vi "Test Restore Point.vi"() -> ()   [LabVIEW 2020, in "Test Executive.lvlib"]
uses:
  <vilib>/gpm_packages/@cs/test-executive/Source/Test Executive/Test Executive.lvlib
  <vilib>/gpm_packages/@cs/test-executive/Source/Test Executive/TestExecutive/Test Executive.lvclass
  C:/Program Files/National Instruments/LabVIEW 2020/vi.lib/gpm_packages/@cs/test-executive/Source/Test Executive/ITestExecutive/ITest Executive.lvclass
  <vilib>/gpm_packages/@cs/test-executive/Source/Test Executive/Executioner/Executioner.lvclass
  866dfd19-2fef-4b99-8a4a-1d31d88e504e.vi
  55b154ae-6d03-47ed-abc2-d28db7feda01.vi
  8564ab31-dd3a-4968-8861-3b4339f4920d.vi
  9b79477b-4d99-41b4-a2fb-9df7ea8afb31.vi
  95889fa5-b0fb-411b-bc35-b648c597537f.vi
  6decda23-fb0c-4e77-ad71-e1f71655b843.vi
  71592cda-0d0e-4ea7-b138-086424aed341.vi
  0583369c-d912-4d49-be3f-0b23069dcf00.vi
  bffa5b7c-ecbc-40cd-a0d5-f9da2a76cf50.vi
  <vilib>/Utility/error.llb/Error Cluster From Error Code.vi
  <vilib>/gpm_packages/@cs/test-executive/Source/Test Executive/ITestExecutive/ITest Executive.lvclass
  <vilib>/gpm_packages/@cs/test-executive/Source/Test Executive/TestExecutive Ref/TestExecutive Ref.lvclass
  c9edba23-499d-4d6b-bf99-6c37c6a75b36.vi
  b25967a6-4fd7-4e76-b6fa-60230ccf68d8.vi
panel:
  out "After Restore Run":string[](array[string])
  in  "Stop final run":bool
  out "Final Run classes":string
  out "Restore Traverse":string[](array[string])
  out "Restore Traverse Classes":string
  in  "stop restore":bool
  out "First Run Array":string[](array[string])
  out "Class":string
  out "Tag":i32
  out "Name":string
  out "Attribute 2":i32
  out "class name":string
  in  "stop":bool
  out "error out":errorcluster
  in  "Test Exec":string(tree)
  out "Pointer?":bool
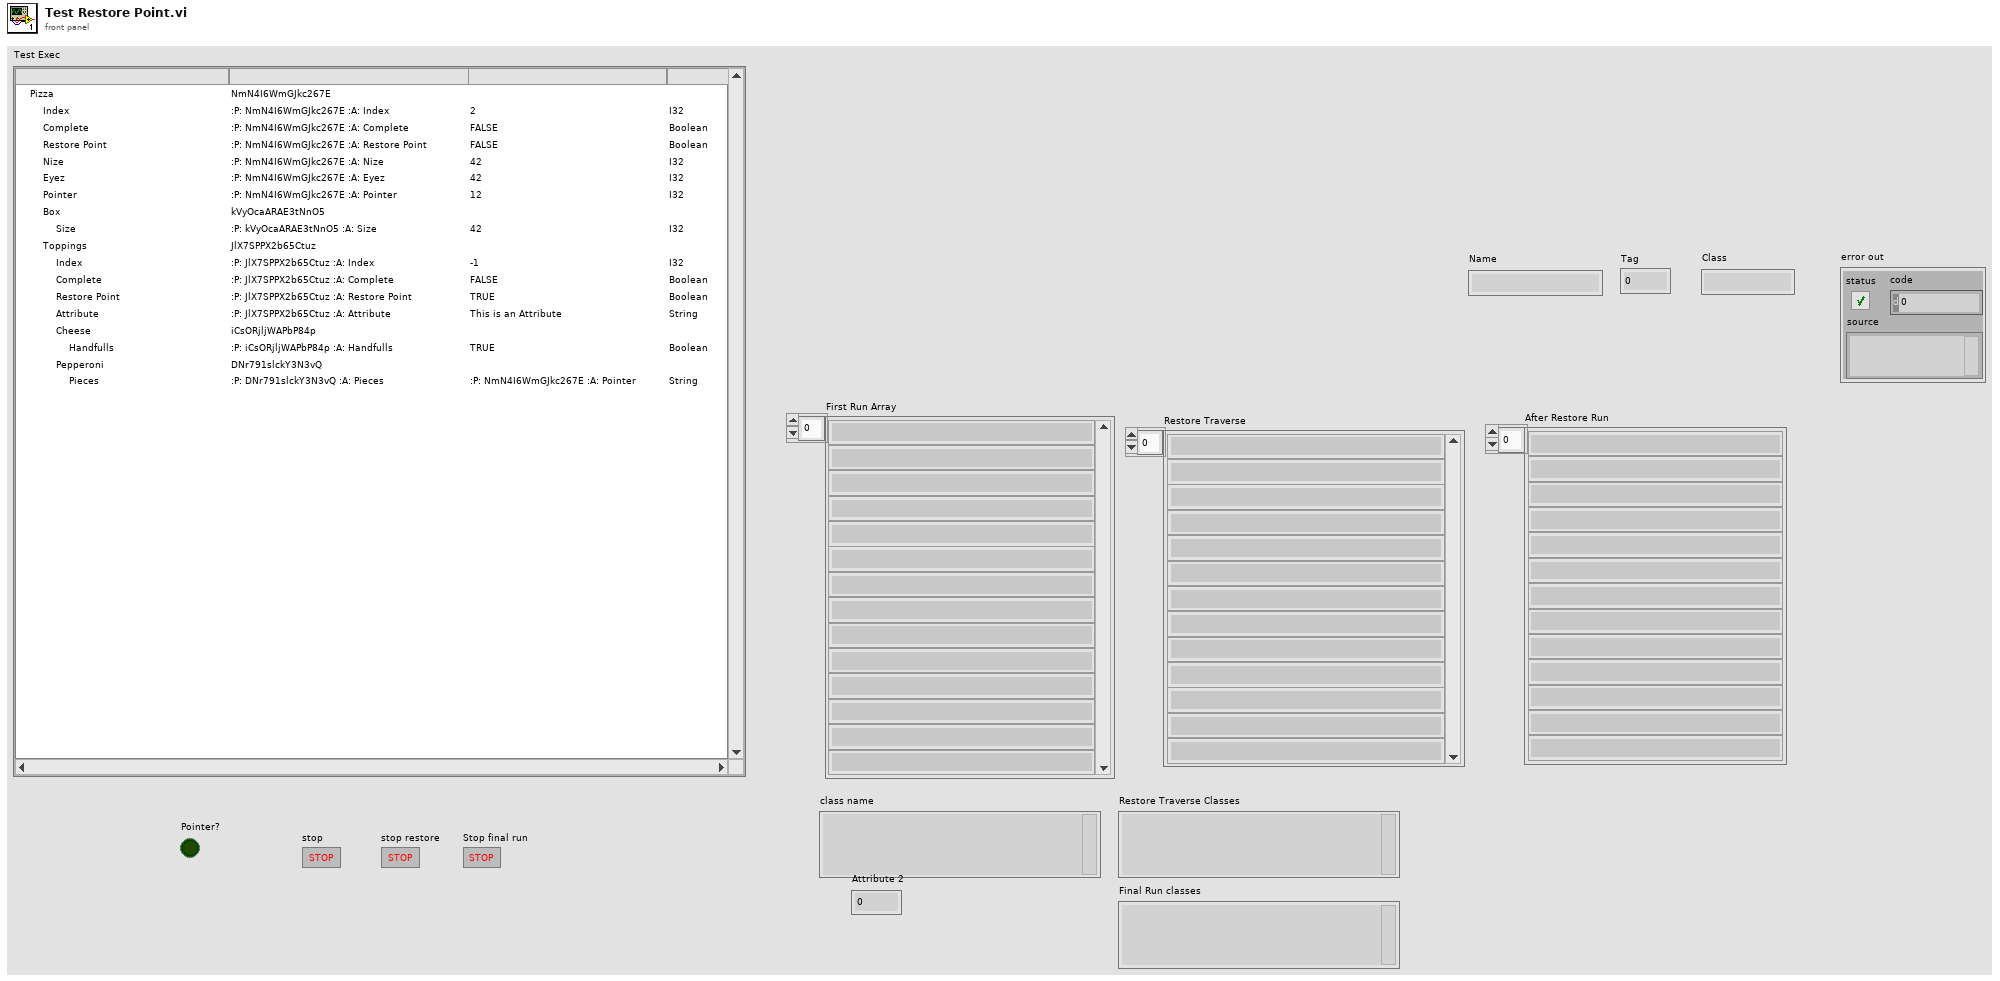
[diagram p1: front panel]
types:
  T1 = cluster{"Left Cell String":string, "Child Text":string[], "Child Tag":string, "Item Indent":i32, "Child Only?":bool, "Glyph Index":i32}[]
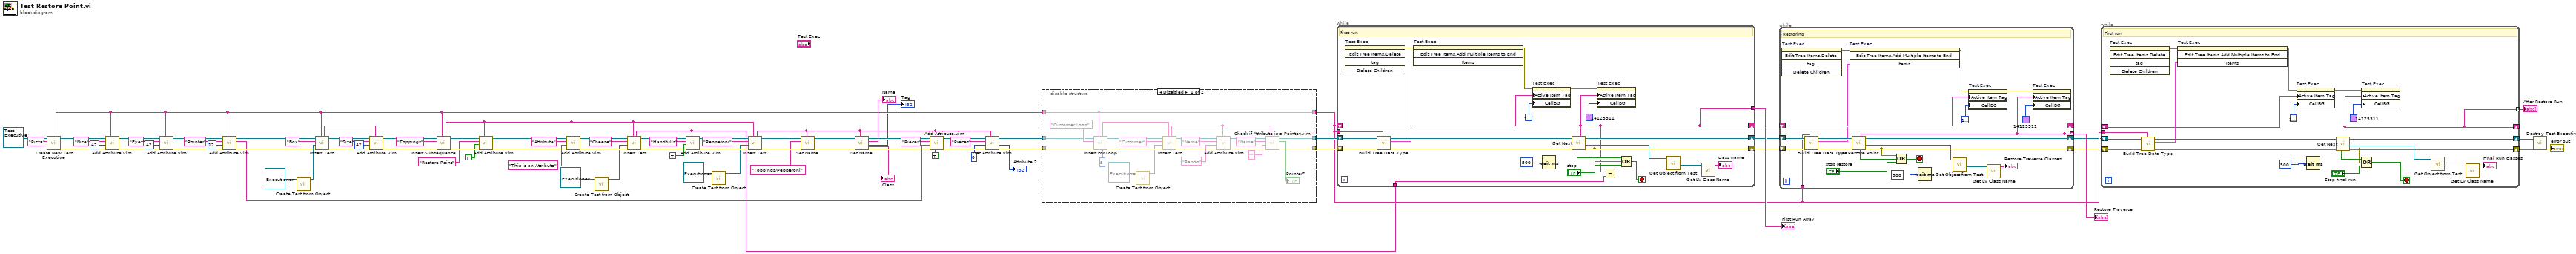
[diagram p0: block diagram]
diagram:
  n1 = call <vilib>:"Create New Test Executive.vi"("Name"="Pizza", "Test Executive"=refnum<class "Test Executive.lvclass"> refnum ("Test Executive.lvlib:Test Executive.lvclass")) -> ("error out"=w56:errorcluster, "Test Executive Ref"=w57:refnum<data-value>, "Test Executive ID out"=w43:string)  [unwired: 7 in]
  n2 = call "Add Attribute.vim"("ID"=w43, "error in (no error)"=w56, "Attribute"=42, "Attribute Name"="Nize", "Test Executive Ref"=w57) -> ("error out"=w52:errorcluster, "Test Executive Ref out"=w53:refnum<data-value>)  [unwired: 3 in, 2 out]
  n3 = call "Add Attribute.vim"("ID"=w43, "error in (no error)"=w52, "Attribute"=42, "Attribute Name"="Eyez", "Test Executive Ref"=w53) -> ("error out"=w47:errorcluster, "Test Executive Ref out"=w45:refnum<data-value>)  [unwired: 3 in, 2 out]
  n4 = call "Add Attribute.vim"("ID"=w43, "error in (no error)"=w47, "Attribute"=12, "Attribute Name"="Pointer", "Test Executive Ref"=w45) -> ("error out"=w46:errorcluster, "Attribute ID out"=w42:string, "Test Executive Ref out"=w44:refnum<data-value>)  [unwired: 3 in, 1 out]
  n5 = call <vilib>:"Create Test from Object.vi"("Test"=refnum<class "Executioner.lvclass"> refnum ("Test Executive.lvlib:Executioner.lvclass")) -> ("Test"=w62:refnum<class "Executioner.lvclass">)  [unwired: 10 in]
  n6 = call <vilib>:"Insert Test.vi"("Parent ID"=w43, "error in (no error)"=w46, "Test"=w62, "Name"="Box", "Test Executive Ref"=w44) -> ("error out"=w70:errorcluster, "Test Executive Ref out"=w85:refnum<data-value>, "Unique ID out"=w84:string)  [unwired: 3 in, 1 out]
  n7 = call "Add Attribute.vim"("ID"=w84, "error in (no error)"=w70, "Attribute"=42, "Attribute Name"="Size", "Test Executive Ref"=w85) -> ("error out"=w50:errorcluster, "Test Executive Ref out"=w51:refnum<data-value>)  [unwired: 3 in, 2 out]
  n8 = call <vilib>:"Insert Subsequence.vi"("Parent ID"=w43, "error in (no error)"=w50, "Name"="Toppings", "Test Executive Ref"=w51) -> ("error out"=w6:errorcluster, "Test Executive Ref out"=w8:refnum<data-value>, "Unique ID out"=w4:string)  [unwired: 4 in, 1 out]
  n9 = call "Add Attribute.vim"("ID"=w4, "error in (no error)"=w6, "Attribute"=TRUE, "Attribute Name"="Restore Point", "Test Executive Ref"=w8) -> ("error out"=w5:errorcluster, "Test Executive Ref out"=w7:refnum<data-value>)  [unwired: 3 in, 2 out]
  n10 = call "Add Attribute.vim"("ID"=w4, "error in (no error)"=w5, "Attribute"="This is an Attribute", "Attribute Name"="Attribute", "Test Executive Ref"=w7) -> ("error out"=w69:errorcluster, "Test Executive Ref out"=w73:refnum<data-value>)  [unwired: 3 in, 2 out]
  n11 = call <vilib>:"Create Test from Object.vi"("Test"=refnum<class "Executioner.lvclass"> refnum ("Test Executive.lvlib:Executioner.lvclass")) -> ("Test"=w64:refnum<class "Executioner.lvclass">)  [unwired: 10 in]
  n12 = call <vilib>:"Insert Test.vi"("Parent ID"=w4, "error in (no error)"=w69, "Test"=w64, "Name"="Cheese", "Test Executive Ref"=w73) -> ("error out"=w68:errorcluster, "Test Executive Ref out"=w79:refnum<data-value>, "Unique ID out"=w1:string)  [unwired: 3 in, 1 out]
  n13 = call "Add Attribute.vim"("ID"=w1, "error in (no error)"=w68, "Attribute"=TRUE, "Attribute Name"="Handfulls", "Test Executive Ref"=w79) -> ("error out"=w67:errorcluster, "Test Executive Ref out"=w74:refnum<data-value>)  [unwired: 3 in, 2 out]
  n14 = call <vilib>:"Create Test from Object.vi"("Test"=refnum<class "Executioner.lvclass"> refnum ("Test Executive.lvlib:Executioner.lvclass")) -> ("Test"=w60:refnum<class "Executioner.lvclass">)  [unwired: 10 in]
  n15 = call <vilib>:"Insert Test.vi"("Parent ID"=w4, "error in (no error)"=w67, "Test"=w60, "Name"="Pepperoni", "Test Executive Ref"=w74) -> ("error out"=w26:errorcluster, "Test Executive Ref out"=w28:refnum<data-value>, "Unique ID out"=w24:string)  [unwired: 3 in, 1 out]
  n16 = call <vilib>:"Set Name.vi"("Unique ID"=w24, "error in (no error)"=w26, "Name"="Toppings/Pepperoni", "Test Executive Ref"=w28) -> ("error out"=w25:errorcluster, "Test Executive Ref out"=w27:refnum<data-value>)  [unwired: 6 in]
  n17 = call <vilib>:"Get Name.vi"("Unique ID"=w24, "error in (no error)"=w25, "Test Executive Ref"=w27) -> ("error out"=w32:errorcluster, "Tag"=→"Tag":i32, "Name"=→"Name":string, "Test Executive Ref out"=w33:refnum<data-value>, "Class"=→"Class":string)  [unwired: 4 in]
  n18 = call "Add Attribute.vim"("Pointer?"=TRUE, "ID"=w24, "error in (no error)"=w32, "Attribute"=w42, "Attribute Name"="Pieces", "Test Executive Ref"=w33) -> ("error out"=w38:errorcluster, "Test Executive Ref out"=w40:refnum<data-value>)  [unwired: 2 in, 2 out]
  n19 = call "Get Attribute.vim"("ID"=w24, "error in (no error)"=w38, "Type"=0, "Attribute Name"="Pieces", "Test Executive Ref"=w40) -> ("error out"=w37:errorcluster, "Attribute"=→"Attribute 2":i32, "Test Executive Ref out"=w39:refnum<data-value>)  [unwired: 2 in, 2 out]
  n20 = disable-structure shown="Disabled" {
    disable-tunnel: w43 -> [w89 w112]
    disable-tunnel: w39 -> [w93 w114]
    disable-tunnel: w37 -> [w92 w113]
    disable-tunnel: [w91 w113] -> w22
    disable-tunnel: [w90 w114] -> w21
    disable-tunnel: [w89 w112] -> w14
    frame Disabled {
      n21 = call <vilib>:"Insert For Loop.vi"("Loop Iterations"=5, "Parent ID"=w89, "error in (no error)"=w92, "Name"="Customer Loop" ("Unique ID"), "Test Executive Ref"=w93) -> ("error out"=w100:errorcluster, "Test Executive Ref out"=w101:refnum<data-value>, "Unique ID out"=w94:string)  [unwired: 3 in, 1 out]
      n22 = call <vilib>:"Create Test from Object.vi"("Test"=refnum<class "Executioner.lvclass"> refnum ("Test Executive.lvlib:Executioner.lvclass")) -> ("Test"=w95:refnum<class "Executioner.lvclass">)  [unwired: 10 in]
      n23 = call <vilib>:"Insert Test.vi"("Parent ID"=w94, "error in (no error)"=w100, "Test"=w95, "Name"="Customer", "Test Executive Ref"=w101) -> ("error out"=w102:errorcluster, "Test Executive Ref out"=w109:refnum<data-value>, "Unique ID out"=w97:string)  [unwired: 3 in, 1 out]
      n24 = call "Add Attribute.vim"("ID"=w97, "error in (no error)"=w102, "Attribute"="Rando", "Attribute Name"="Name", "Test Executive Ref"=w109) -> ("error out"=w106:errorcluster, "Test Executive Ref out"=w107:refnum<data-value>)  [unwired: 3 in, 2 out]
      n25 = call "Check if Attribute is a Pointer.vim"("ID"=w97, "error in (no error)"=w106, "Type"="", "Attribute Name"="Name", "Test Executive Ref"=w107) -> ("error out"=w91:errorcluster, "Pointer?"=→"Pointer?":bool, "Test Executive Ref out"=w90:refnum<data-value>)  [unwired: 2 in, 2 out]
    }
    frame Enabled {
    }
  }
  n26 = while {
    shift-right: [w137] -> w19
    shift-left: w21 -> [w126]
    shift-right: [w135] -> w18
    shift-left: w22 -> [w125]
    shift-right: [w116] -> w17
    shift-left: w14 -> [w119]
    tunnel: [w116] -> w20 mode=indexing
    tunnel: w14 -> [w118]
    tunnel: w1 -> [w115]
    stop <- w133 stop-if-true
    # "First run"
    n27 = invoke on="Test Exec" class="Tree (strict)" method="Edit Tree Items.Delete"() -> (error out=w117:errorcluster)  [unwired: 5 in, 4 out]
    n28 = call <vilib>:"Build Tree Data Type.vi"("Test ID"=w118, "error in (no error)"=w125, "Test Executive Ref"=w126) -> ("error out"=w124:errorcluster, "Tree Data"=w122:T1, "Test Executive Ref out"=w123:refnum<data-value>)  [unwired: 6 in]
    n29 = invoke on="Test Exec" class="Tree (strict)" method="Edit Tree Items.Add Multiple Items to End"(error in=w117, "Items"=w122) -> (error out=w121:errorcluster)  [unwired: 2 in, 3 out]
    n30 = property on="Test Exec" class="Tree (strict)"(error in=w121, "Active Item Tag"=w119, "CellBG"=u32 16777226) -> (error out=w120:errorcluster)  [unwired: 1 in, 1 out]
    n31 = Wait (ms)(milliseconds to wait=u32 500) -> ()  [unwired: 1 out]
    n32 = call <vilib>:"Get Next.vi"("error in (no error)"=w124, "Test Executive Ref"=w123) -> ("error out"=w135:errorcluster, "Test"=w129:refnum<class "Executioner.lvclass">, "Test Executive Ref out"=w137:refnum<data-value>, "Unique ID out"=w116:string, "Complete"=w136:bool)  [unwired: 3 in, 2 out]
    n33 = property on="Test Exec" class="Tree (strict)"(error in=w120, "Active Item Tag"=w116, "CellBG"=u32 14125311) -> ()  [unwired: 1 in, 2 out]
    n34 = Equal?(x=w116, y=w115) -> ()  [unwired: 1 out]
    n35 = Compound Arithmetic op=OR(w136, w135, "stop") -> (w133:bool)
    n36 = call <vilib>:"Get Object from Test.vi"("Executioner in"=w129) -> ("Test"=w128:refnum<class>)  [unwired: 9 in, 1 out]
    n37 = call <vilib>:"Get LV Class Name.vi"("object"=w128) -> ("class name"=→"class name":string)  [unwired: 9 in, 1 out]
  }
  "First Run Array" <- w20
  n38 = while {
    tunnel: w14 -> [w155]
    shift-right: [w141] -> w15
    shift-left: w17 -> [w149]
    tunnel: [w141] -> w16 mode=indexing
    shift-right: [w139] -> w12
    shift-left: w19 -> [w159]
    shift-right: [w138] -> w13
    shift-left: w18 -> [w158]
    stop <- w142 stop-if-true
    # "Restoring"
    n39 = invoke on="Test Exec" class="Tree (strict)" method="Edit Tree Items.Delete"() -> (error out=w154:errorcluster)  [unwired: 5 in, 4 out]
    n40 = call <vilib>:"Build Tree Data Type.vi"("Test ID"=w155, "error in (no error)"=w158, "Test Executive Ref"=w159) -> ("error out"=w157:errorcluster, "Tree Data"=w140:T1, "Test Executive Ref out"=w156:refnum<data-value>)  [unwired: 6 in]
    n41 = invoke on="Test Exec" class="Tree (strict)" method="Edit Tree Items.Add Multiple Items to End"(error in=w154, "Items"=w140) -> (error out=w152:errorcluster)  [unwired: 2 in, 3 out]
    n42 = call <vilib>:"Get Restore Point.vi"("error in (no error)"=w157, "Test Executive Ref"=w156) -> ("error out"=w138:errorcluster, "Test"=w144:refnum<class "Executioner.lvclass">, "Test Executive Ref out"=w139:refnum<data-value>, "Restore Point"=w147:bool, "Unique ID out"=w141:string)  [unwired: 4 in, 1 out]
    n43 = Compound Arithmetic op=OR(w138, w147, "stop restore") -> (w142:bool)
    n44 = Wait (ms)(milliseconds to wait=u32 500) -> ()  [unwired: 1 out]
    n45 = call <vilib>:"Get Object from Test.vi"("Executioner in"=w144) -> ("Test"=w145:refnum<class>)  [unwired: 9 in, 1 out]
    n46 = property on="Test Exec" class="Tree (strict)"(error in=w152, "Active Item Tag"=w149, "CellBG"=u32 16777226) -> (error out=w153:errorcluster)  [unwired: 1 in, 1 out]
    n47 = call <vilib>:"Get LV Class Name.vi"("object"=w145) -> ("class name"=→"Restore Traverse Classes":string)  [unwired: 9 in, 1 out]
    n48 = property on="Test Exec" class="Tree (strict)"(error in=w153, "Active Item Tag"=w141, "CellBG"=u32 14125311) -> ()  [unwired: 1 in, 2 out]
  }
  "Restore Traverse" <- w16
  n49 = while {
    shift-right: [w181] -> w11
    shift-left: w12 -> [w170]
    shift-right: [w179] -> w10
    shift-left: w13 -> [w169]
    shift-right: [w165] -> _
    shift-left: w15 -> [w162]
    tunnel: [w165] -> w9 mode=indexing
    tunnel: w14 -> [w161]
    stop <- w177 stop-if-true
    # "First run"
    n50 = invoke on="Test Exec" class="Tree (strict)" method="Edit Tree Items.Delete"() -> (error out=w160:errorcluster)  [unwired: 5 in, 4 out]
    n51 = call <vilib>:"Build Tree Data Type.vi"("Test ID"=w161, "error in (no error)"=w169, "Test Executive Ref"=w170) -> ("error out"=w168:errorcluster, "Tree Data"=w166:T1, "Test Executive Ref out"=w167:refnum<data-value>)  [unwired: 6 in]
    n52 = invoke on="Test Exec" class="Tree (strict)" method="Edit Tree Items.Add Multiple Items to End"(error in=w160, "Items"=w166) -> (error out=w164:errorcluster)  [unwired: 2 in, 3 out]
    n53 = property on="Test Exec" class="Tree (strict)"(error in=w164, "Active Item Tag"=w162, "CellBG"=u32 16777226) -> (error out=w163:errorcluster)  [unwired: 1 in, 1 out]
    n54 = Wait (ms)(milliseconds to wait=u32 500) -> ()  [unwired: 1 out]
    n55 = call <vilib>:"Get Next.vi"("error in (no error)"=w168, "Test Executive Ref"=w167) -> ("error out"=w179:errorcluster, "Test"=w173:refnum<class "Executioner.lvclass">, "Test Executive Ref out"=w181:refnum<data-value>, "Unique ID out"=w165:string, "Complete"=w180:bool)  [unwired: 3 in, 2 out]
    n56 = property on="Test Exec" class="Tree (strict)"(error in=w163, "Active Item Tag"=w165, "CellBG"=u32 14125311) -> ()  [unwired: 1 in, 2 out]
    n57 = Compound Arithmetic op=OR(w180, w179, "Stop final run") -> (w177:bool)
    n58 = call <vilib>:"Get Object from Test.vi"("Executioner in"=w173) -> ("Test"=w172:refnum<class>)  [unwired: 9 in, 1 out]
    n59 = call <vilib>:"Get LV Class Name.vi"("object"=w172) -> ("class name"=→"Final Run classes":string)  [unwired: 9 in, 1 out]
  }
  "After Restore Run" <- w9
  n60 = call <vilib>:"Destroy Test Executive.vi"("error in (no error)"=w10, "Test Executive Ref"=w11) -> ("error out"=→"error out":errorcluster)  [unwired: 9 in]
